vi "PXI-Find Devices.vi"(11 "error in (no error)":errorcluster) -> (4 "Num AO":i32[](array[numeric]), 6 "Num AI":i32[](array[numeric]), 8 "Slot Num":u32[](array[numeric]), 15 "error out":errorcluster)   [LabVIEW 2020]
uses:
  <resource>/objmgr/daqmx.rc
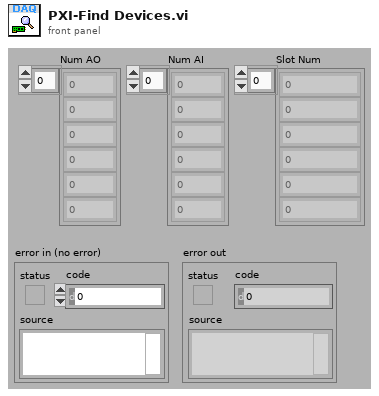
[diagram p1: front panel]
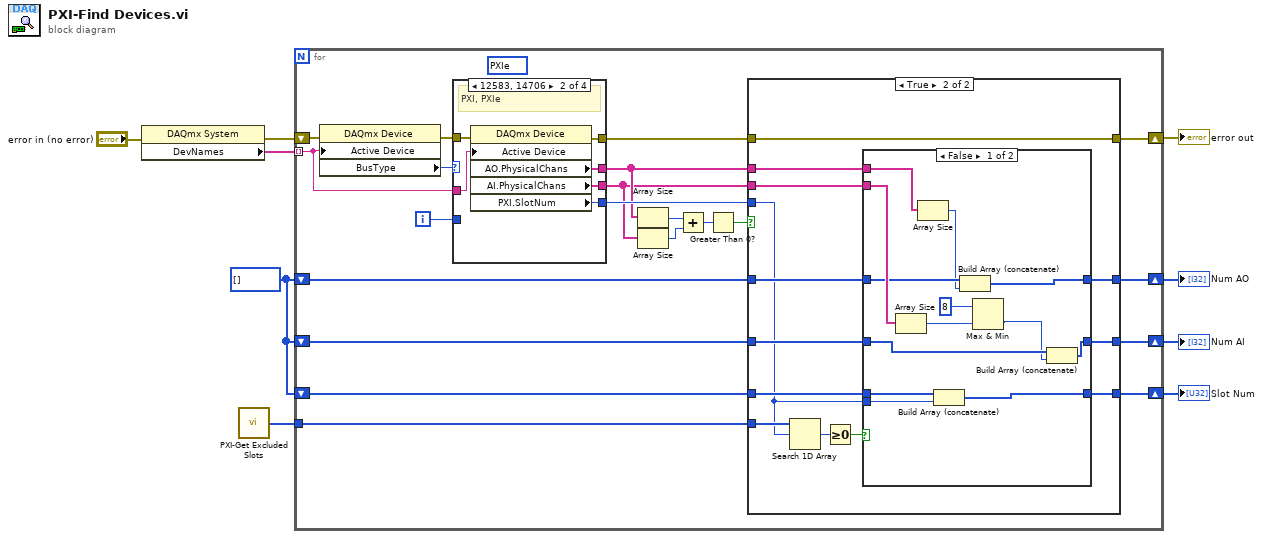
[diagram p0: block diagram]
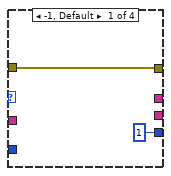
[diagram p4: hidden frame]
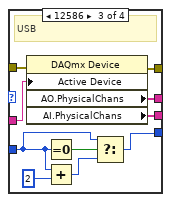
[diagram p5: hidden frame]
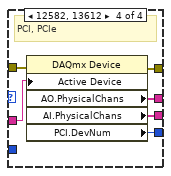
[diagram p6: hidden frame]
diagram:
  w1 = i32[] [] ("Num AO")
  n1 = property class="DAQmx System"(error in="error in (no error)") -> (error out=w7:errorcluster, "DevNames"=w8:tag[])  [unwired: 1 in, 1 out]
  n2 = call "PXI-Get Excluded Slots.vi"() -> ("excluded slots"=w2:i32[])  [unwired: 14 in, 1 out]
  n3 = for {
    tunnel: w8 -> [w20] mode=indexing
    shift-right: [w17] -> w6
    shift-left: w7 -> [w23]
    tunnel: w2 -> [w29]
    shift-right: [w30] -> w5
    shift-left: w1 -> [w26]
    shift-right: [w24] -> w4
    shift-left: w1 -> [w25]
    shift-right: [w27] -> w3
    shift-left: w1 -> [w28]
    i -> [w19]
    (unwired) 14706 items=["PCI"=12582, "PCIe"=13612, "PXI"=12583, "PXIe"=14706, "SCXI"=12584, "SCC"=14707, "PCCard"=12585, "USB"=12586, "CompactDAQ"=14637, "TCP/IP"=14828, "Unknown"=12588, "SwitchBlock"=15870] ("BusType")
    n4 = property class="DAQmx Device"(error in=w23, "Active Device"=w20) -> (error out=w22:errorcluster, "BusType"=w21:i32)  [unwired: 1 in, 1 out]
    n5 = case shown="12583, 14706" w21 {
      tunnel: [_ w71 w81 w87] -> w15
      tunnel: [_ w70 w80 w86] -> w14
      tunnel: [w65 w69 w79 w85] -> w18
      tunnel: [u32 1 ("PCI.DevNum") w68 w75 w84] -> w16
      tunnel: w22 -> [w65 w67 w78 w83]
      tunnel: w20 -> [_ w66 w77 w82]
      tunnel: w19 -> [_ _ w74 _]
      frame -1, Default {
      }
      frame 12583, 14706 {
        # "PXI, PXIe"
        n6 = property class="DAQmx Device"(error in=w67, "Active Device"=w66) -> (error out=w69:errorcluster, "AO.PhysicalChans"=w71:tag[], "AI.PhysicalChans"=w70:tag[], "PXI.SlotNum"=w68:u32)  [unwired: 1 in, 1 out]
      }
      frame 12586 {
        # "USB"
        n7 = property class="DAQmx Device"(error in=w78, "Active Device"=w77) -> (error out=w79:errorcluster, "AO.PhysicalChans"=w81:tag[], "AI.PhysicalChans"=w80:tag[])  [unwired: 1 in, 1 out]
        n8 = Equal To 0?(x=w74) -> (x = 0?=w76:bool)
        n9 = Add(x=w74, y=2) -> (x+y=w73:i32)
        n10 = Select(t=w74, s=w76, f=w73) -> (s? t:f=w75:i32)
      }
      frame 12582, 13612 {
        # "PCI, PCIe"
        n11 = property class="DAQmx Device"(error in=w83, "Active Device"=w82) -> (error out=w85:errorcluster, "AO.PhysicalChans"=w87:tag[], "AI.PhysicalChans"=w86:tag[], "PCI.DevNum"=w84:u32)  [unwired: 1 in, 1 out]
      }
    }
    n12 = Array Size(array=w15) -> (size(s)=w12:i32)
    n13 = Array Size(array=w14) -> (size(s)=w11:i32)
    n14 = Add(x=w12, y=w11) -> (x+y=w13:i32)
    n15 = Greater Than 0?(x=w13) -> (x > 0?=w10:bool)
    n16 = case shown="True" w10 {
      tunnel: w15 -> [_ w47]
      tunnel: [w33 w46] -> w30
      tunnel: w14 -> [_ w45]
      tunnel: w29 -> [_ w44]
      tunnel: w28 -> [w31 w42]
      tunnel: [w31 w41] -> w27
      tunnel: w26 -> [w33 w40]
      tunnel: w25 -> [w32 w38]
      tunnel: [w32 w37] -> w24
      tunnel: w16 -> [_ w36]
      tunnel: w18 -> [w34 w35]
      tunnel: [w34 w35] -> w17
      frame False {
      }
      frame True {
        n17 = Search 1D Array(1D array=w44, element=w36) -> (index of element=w43:i32)  [unwired: 1 in]
        n18 = Greater Or Equal To 0?(x=w43) -> (x >= 0?=w39:bool)
        n19 = case shown="False" w39 {
          tunnel: w47 -> [w60 _]
          tunnel: [w53 w62] -> w46
          tunnel: w45 -> [w59 _]
          tunnel: [w51 w61] -> w37
          tunnel: w42 -> [w58 w63]
          tunnel: w36 -> [w57 _]
          tunnel: [w56 w63] -> w41
          tunnel: w40 -> [w55 w62]
          tunnel: w38 -> [w52 w61]
          frame False {
            n20 = Array Size(array=w59) -> (size(s)=w49:i32)
            n21 = Array Size(array=w60) -> (size(s)=w54:i32)
            n22 = Build Array (concatenate)(w58, w57) -> (w56:u32[])
            n23 = Build Array (concatenate)(w55, w54) -> (w53:i32[])
            n24 = Max & Min(x=8 ("y"), y=w49) -> (min(x,y)=w48:i32)  [unwired: 1 out]
            n25 = Build Array (concatenate)(w52, w48) -> (w51:i32[])
          }
          frame True {
          }
        }
      }
    }
  }
  "error out" <- w6
  "Num AO" <- w5
  "Num AI" <- w4
  "Slot Num" <- w3
